vi "qualify channel.vi"(10 "unqualified channel":refnum<class "TBM channel.lvclass">, 11 "module configuration in":refnum<class "TBM module configuration.lvclass">) -> (2 "qualified channel":refnum<class "TBM channel.lvclass">, 3 "module configuration out":refnum<class "TBM module configuration.lvclass">)   [LabVIEW 2013, in "TBM module configuration.lvclass"]
doc: "Converts an unqualified channel into a qualified channel, based on the rules of the module. A qualified channel id is <module instance id>/<channel id>"
uses:
  TBM module configuration.lvclass
  channel/TBM channel.lvclass
  <vilib>/NI/Tag Bus/tag/tag descriptor.lvclass/tag descriptor.ctl
  <vilib>/NI/Configuration Framework/serializable configuration/NISE_CEF_serializable configuration.lvclass/NISE_CEF_serializable configuration.ctl
  <vilib>/NI/Configuration Framework/serializable configuration/NISE_CEF_serializable configuration.lvclass
  <vilib>/NI/Tag Bus/tag/tag descriptor.lvclass
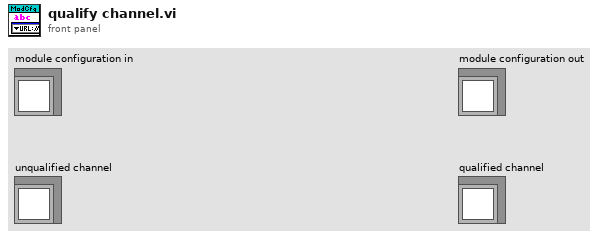
[diagram p1: front panel]
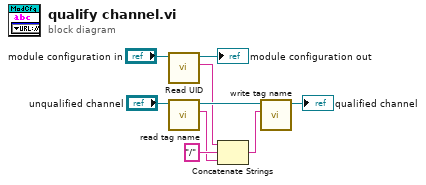
[diagram p0: block diagram]
diagram:
  n1 = call <vilib>:"Read UID.vi"("configuration in"="module configuration in") -> ("instance id"=w3:string, "configuration out"=→"module configuration out":refnum<class "TBM module configuration.lvclass">)  [unwired: 8 in, 1 out]
  n2 = call <vilib>:"read tag name.vi"("system tag in"="unqualified channel") -> ("name"=w7:string, "system tag out"=w6:refnum<class "TBM channel.lvclass">)  [unwired: 8 in, 1 out]
  n3 = Concatenate Strings(w3, "/" ("string"), w7) -> (w9:string)
  n4 = call <vilib>:"write tag name.vi"("name"=w9, "system tag in"=w6) -> ("system tag out"=→"qualified channel":refnum<class "TBM channel.lvclass">)  [unwired: 8 in, 1 out]
